vi "Stepper_stage_test.vi"() -> ()   [LabVIEW 2019]
uses:
  <vilib>/FPGAPlugInAG/myRIO-1900/niLvFpga_Open_myRIO-1900.vi
  <vilib>/rvi/interface/common/dynamic/niFpgaDynamicAddResources.vi
  <vilib>/Utility/error.llb/Error Cluster From Error Code.vi
  <vilib>/rvi/errors/niLvFpgaAdjustHostInterfaceError.vi
  <vilib>/FPGAPlugInAG/Dynamic/niLvFpga_Close_Dynamic.vi
  <vilib>/rvi/interface/nirviOpenFPGA/nirviOpenFPGA.xnode
  FPGA Bitfiles/encodertest_FPGATarget_PPGAdriver_bE+majGn1xs.lvbitx
  <vilib>/rvi/interface/nirviReadWriteControl/nirviReadWriteControl.xnode
  <vilib>/rvi/interface/nirviCloseFPGA/nirviCloseFPGA.xnode
  <vilib>/rvi/interface/Simulation/niFpgaSimulationCallBeginRW.vi
  NiFpgaLv.dll
panel:
  in  "Stop":bool
  in  "ENABLE":bool
  in  "Position Loop \nPeriod (ms)":u32=2
  in  "Position\nCommand":i32
  in  "Gear Ratio":i32=4
  in  "SubSteps/FullStep":i32=16
  in  "Speed Limit\n[Rotations/s]":dbl=5.0
  in  "FWD/BCK":bool
  in  "Move":bool
  out "error out":errorcluster
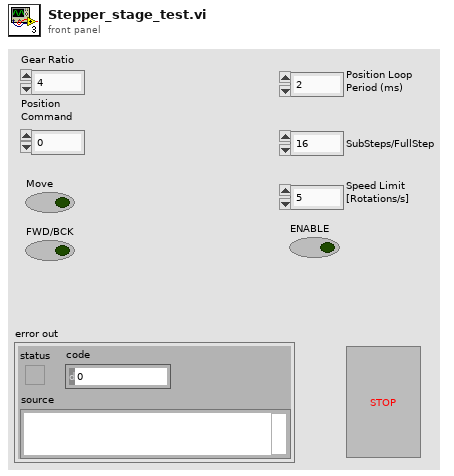
[diagram p1: front panel]
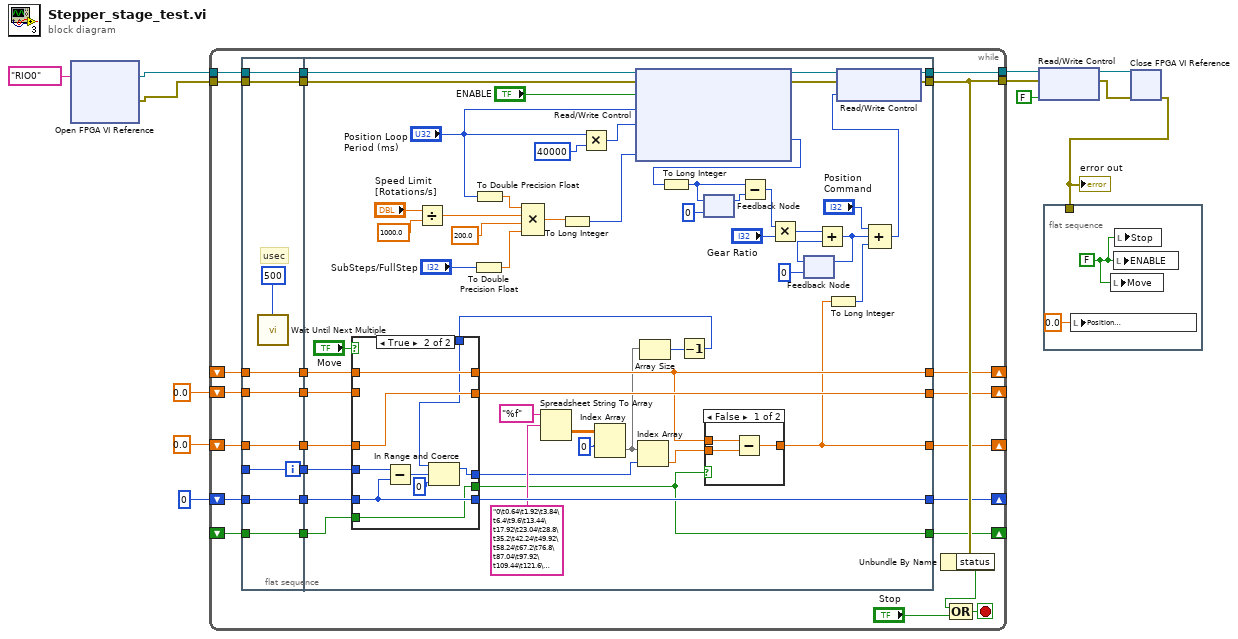
[diagram p0: block diagram]
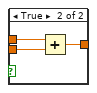
[diagram p2: hidden frame]
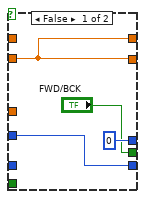
[diagram p3: hidden frame]
diagram:
  n1 = xnode "Open FPGA VI Reference"("resource name"=tag "RIO0") -> ("FPGA VI Reference Out"=w3:refnum<k20>, "error out"=w2:errorcluster)  [unwired: 1 in]
  n2 = while {
    tunnel: [w35] -> w12
    tunnel: [w34] -> w11
    tunnel: w3 -> [w37]
    tunnel: w2 -> [w36]
    shift-right: [w32] -> _
    shift-left: 0 -> [w30]
    shift-right: [w21] -> _
    shift-left: 0.0 -> [w29]
    shift-right: [w27] -> _
    shift-left: 0.0 -> [w28]
    shift-right: [w25] -> _
    shift-left: _ -> [w26]
    shift-right: [w24] -> _
    shift-left: _ -> [w23]
    i -> [w31]
    stop <- w22 stop-if-true
    n3 = flat-sequence {
      tunnel: w23 -> [w40]
      tunnel: w26 -> [w41]
      tunnel: w28 -> [w42]
      tunnel: w29 -> [w43]
      tunnel: w30 -> [w44]
      tunnel: w31 -> [w45]
      tunnel: w36 -> [w46]
      tunnel: w37 -> [w47]
      tunnel: [w47] -> w20
      tunnel: [w46] -> w19
      tunnel: [w45] -> w18
      tunnel: [w44] -> w17
      tunnel: [w43] -> w16
      tunnel: [w42] -> w15
      tunnel: [w41] -> w14
      tunnel: [w40] -> w13
      tunnel: [w94] -> w35
      tunnel: [w93] -> w34
      tunnel: [w71] -> w32
      tunnel: [w66] -> w27
      tunnel: [w62] -> w25
      tunnel: [w54] -> w24
      tunnel: [w50] -> w21
      tunnel: w20 -> [w100]
      tunnel: w19 -> [w98]
      tunnel: w18 -> [w70]
      tunnel: w17 -> [w69]
      tunnel: w16 -> [w68]
      tunnel: w15 -> [w67]
      tunnel: w14 -> [w63]
      tunnel: w13 -> [w53]
      frame #0 {
        # "usec"
        n4 = call "Wait Until Next Multiple"("Count(uSec)"=u32 500 ("millisecond multiple")) -> ()  [unwired: 1 out]
      }
      frame #1 {
        n5 = Divide(x="Speed Limit\n[Rotations/s]", y=1000.0) -> (x/y=w80:dbl)
        n6 = To Double Precision Float(number="SubSteps/FullStep") -> (double precision float=w75:dbl)
        n7 = To Double Precision Float(number="Position Loop \nPeriod (ms)") -> (double precision float=w74:dbl)
        n8 = Compound Arithmetic op=MULTIPLY(w74, w80, 200.0 ("value"), w75) -> (w78:dbl)
        n9 = Spreadsheet String To Array(format string="%f", spreadsheet string="0\t0.64\t1.92\t3.84\t6.4\t9.6\t13.44\t17.92\t23.04\t28.8\t35.2\t42.24\t49.92\t58.24\t67.2\t76.8\t87.04\t97.92\t109.44\t121.6\t134.4\t147.84\t161.92\t176.64\t192\t208\t224.64\t241.92\t259.84\t278.4\t297.6\t317.44\t337.92\t359.04\t380.8\t403.2\t426.24\t449.92\t474.24\t499.2\t524.8\t551.04\t577.92\t605.44\t633.6\t662.4\t691.84\t721.92\t752.64\t784\t816\t848.64\t881.92\t915.84\t950.4\t985.6\t1021.4\t1057.9\t1095\t1132.8\t1171.2\t1210.2\t1249.9\t1290.2\t1331.2\t1372.8\t1415\t1457.9\t1501.4\t1545.6\t1590.4\t1635.8\t1681.9\t1728.6\t1776\t1824\t1872.6\t1921.9\t1971.8\t2022.4\t2073.6\t2125.4\t2177.9\t2231\t2284.8\t2339.2\t2394.2\t2449.9\t2506.2\t2563.2\t2620.8\t2679\t2737.9\t2797.4\t2857.6\t2918.4\t2979.8\t3041.9\t3104.6\t3168\t3232\t3296.6\t3361.9\t3427.8\t3494.4\t3561.6\t3629.4\t3697.9\t3767\t3836.8\t3907.2\t3978.2\t4049.9\t4122.2\t4195.2\t4268.8\t4343\t4417.9\t4493.4\t4569.6\t4646.4\t4723.8\t4801.9\t4880.6\t4960\t5040\t5120.6\t5201.9\t5283.8\t5366.4\t5449.6\t5533.4\t5617.9\t5703\t5788.8\t5875.2\t5962.2\t6049.9\t6138.2\t6227.2\t6316.8\t6407\t6497.9\t6589.4\t6681.6\t6774.4\t6867.8\t6961.9\t7056.6\t7152\t7248\t7344.6\t7441.9\t7539.8\t7638.4\t7737.6\t7837.4\t7937.9\t8039\t8140.8\t8243.2\t8346.2\t8449.9\t8554.2\t8659.2\t8764.8\t8871\t8977.9\t9085.4\t9193.6\t9302.4\t9411.8\t9521.9\t9632.6\t9744\t9856\t9968.6\t10082\t10196\t10310\t10426\t10541\t10658\t10775\t10893\t11011\t11130\t11250\t11370\t11491\t11613\t11735\t11858\t11981\t12106\t12230\t12356\t12482\t12609\t12736\t12864\t12993\t13122\t13252\t13382\t13514\t13645\t13778\t13911\t14045\t14179\t14314\t14450\t14586\t14723\t14861\t14999\t15138\t15277\t15418\t15558\t15700\t15842\t15985\t16128\t16272\t16417\t16562\t16708\t16854\t17002\t17149\t17298\t17447\t17597\t17747\t17898\t18050\t18202\t18355\t18509\t18663\t18818\t18973\t19130\t19286\t19444\t19602\t19761\t19920\t20080\t20240\t20400\t20560\t20720\t20880\t21040\t21200\t21360\t21520\t21680\t21840\t22000\t22160\t22320\t22480\t22640\t22800\t22960\t23120\t23280\t23440\t23600\t23760\t23920\t24080\t24240\t24400\t24560\t24720\t24880\t25040\t25200\t25360\t25520\t25680\t25840\t26000\t26160\t26320\t26480\t26640\t26800\t26960\t27120\t27280\t27440\t27600\t27760\t27920\t28080\t28240\t28399\t28558\t28716\t28874\t29030\t29187\t29342\t29497\t29651\t29805\t29958\t30110\t30262\t30413\t30563\t30713\t30862\t31011\t31158\t31306\t31452\t31598\t31743\t31888\t32032\t32175\t32318\t32460\t32602\t32742\t32883\t33022\t33161\t33299\t33437\t33574\t33710\t33846\t33981\t34115\t34249\t34382\t34515\t34646\t34778\t34908\t35038\t35167\t35296\t35424\t35551\t35678\t35804\t35930\t36054\t36179\t36302\t36425\t36547\t36669\t36790\t36910\t37030\t37149\t37267\t37385\t37502\t37619\t37734\t37850\t37964\t38078\t38191\t38304\t38416\t38527\t38638\t38748\t38858\t38966\t39075\t39182\t39289\t39395\t39501\t39606\t39710\t39814\t39917\t40019\t40121\t40222\t40323\t40422\t40522\t40620\t40718\t40815\t40912\t41008\t41103\t41198\t41292\t41386\t41478\t41571\t41662\t41753\t41843\t41933\t42022\t42110\t42198\t42285\t42371\t42457\t42542\t42627\t42710\t42794\t42876\t42958\t43039\t43120\t43200\t43279\t43358\t43436\t43514\t43590\t43667\t43742\t43817\t43891\t43965\t44038\t44110\t44182\t44253\t44323\t44393\t44462\t44531\t44598\t44666\t44732\t44798\t44863\t44928\t44992\t45055\t45118\t45180\t45242\t45302\t45363\t45422\t45481\t45539\t45597\t45654\t45710\t45766\t45821\t45875\t45929\t45982\t46035\t46086\t46138\t46188\t46238\t46287\t46336\t46384\t46431\t46478\t46524\t46570\t46614\t46659\t46702\t46745\t46787\t46829\t46870\t46910\t46950\t46989\t47027\t47065\t47102\t47139\t47174\t47210\t47244\t47278\t47311\t47344\t47376\t47407\t47438\t47468\t47498\t47526\t47555\t47582\t47609\t47635\t47661\t47686\t47710\t47734\t47757\t47779\t47801\t47822\t47843\t47862\t47882\t47900\t47918\t47935\t47952\t47968\t47983\t47998\t48012\t48026\t48038\t48051\t48062\t48073\t48083\t48093\t48102\t48110\t48118\t48125\t48131\t48137\t48142\t48147\t48150\t48154\t48156\t48158\t48159\t48160") -> (array=w60:dbl[][])  [unwired: 2 in]
        n10 = To Long Integer(number=w78) -> (32bit integer=w77:i32)
        n11 = Multiply(x="Position Loop \nPeriod (ms)", y=u32 40000) -> (x*y=w92:u32)
        n12 = Index Array(array=w60, index (row)=0 ("disabled index (col)")) -> (element=w57:dbl[])  [unwired: 1 in]
        n13 = xnode "Read/Write Control"("FPGA VI Reference In"=w100, "error in"=w98, "ENABLE"="ENABLE", "Position Loop Period (ms)"="Position Loop \nPeriod (ms)", "Num Clocks per Period"=w92, "Velocity  Limit"=w77) -> ("FPGA VI Reference Out"=w96:refnum<k20>, "error out"=w95:errorcluster, "Encoder Position"=w90:i16)
        n14 = Array Size(array=w57) -> (size(s)=w56:i32)
        n15 = To Long Integer(number=w90) -> (32bit integer=w88:i32)
        n16 = Decrement(x=w56) -> (x-1=w55:i32)
        n17 = case shown="True" "Move" {
          tunnel: [w110 w118] -> w71
          tunnel: w70 -> [w110 w119]
          tunnel: w69 -> [_ w118]
          tunnel: [0 ("disabled index (col)") w113] -> w58
          tunnel: w68 -> [_ w117]
          tunnel: [w108 w117] -> w66
          tunnel: w67 -> [w108 _]
          tunnel: [w108 w116] -> w62
          tunnel: w63 -> [_ w116]
          tunnel: w55 -> [_ w112]
          tunnel: ["FWD/BCK" w111] -> w54
          tunnel: w53 -> [_ w111]
          frame False {
          }
          frame True {
            n18 = Subtract(x=w119, y=w118) -> (x-y=w115:i32)
            n19 = In Range and Coerce(upper limit=w112, x=w115, lower limit=0) -> (coerced(x)=w113:i32)  [unwired: 1 out]
          }
        }
        n20 = Index Array(array=w57, index=w58) -> (element=w59:dbl)
        n21 = feedback #1(0) -> (w89:i32)
        n22 = feedback-in #1(w88) -> ()
        n23 = case shown="False" w54 {
          tunnel: w59 -> [w102 w106]
          tunnel: [w103 w105] -> w50
          tunnel: w62 -> [w101 w104]
          frame False {
            n24 = Subtract(x=w101, y=w102) -> (x-y=w103:dbl)
          }
          frame True {
            n25 = Add(x=w104, y=w106) -> (x+y=w105:dbl)
          }
        }
        n26 = Subtract(x=w88, y=w89) -> (x-y=w87:i32)
        n27 = Multiply(x=w87, y="Gear Ratio") -> (x*y=w85:i32)
        n28 = feedback #2(0) -> (w83:i32)
        n29 = Add(x=w85, y=w83) -> (x+y=w48:i32)
        n30 = feedback-in #2(w48) -> ()
        n31 = To Long Integer(number=w50) -> (32bit integer=w51:i32)
        n32 = Compound Arithmetic op=ADD("Position\nCommand", w48, w51) -> (w52:i32)
        n33 = xnode "Read/Write Control"("FPGA VI Reference In"=w96, "error in"=w95, "Position Ref."=w52) -> ("FPGA VI Reference Out"=w94:refnum<k20>, "error out"=w93:errorcluster)
      }
    }
    n34 = Unbundle By Name(w34) -> ("status"=w33:bool)
    n35 = Compound Arithmetic op=OR(w33, "Stop") -> (w22:bool)
  }
  n36 = xnode "Read/Write Control"("FPGA VI Reference In"=w12, "error in"=w11, "ENABLE"=FALSE ("Disable Drive")) -> ("FPGA VI Reference Out"=w9:refnum<k20>, "error out"=w8:errorcluster)
  n37 = flat-sequence {
    tunnel: w4 -> [_]
    frame #0 {
      w121 = FALSE ("ENABLE")
      n38 = local write "Position\nCommand"(0.0 ("Position Command")) -> ()
      n39 = local write "Move"(w121) -> ()
      n40 = local write "ENABLE"(w121) -> ()
      n41 = local write "Stop"(w121) -> ()
    }
  }
  n42 = xnode "Close FPGA VI Reference"("FPGA VI Reference In"=w9, "error in"=w8) -> ("error out"=w4:errorcluster)
  "error out" <- w4
